vi "Wiimote Parse Extension Controller.vi"(8 "error in":errorcluster, 11 "pReportBuffer in":u8[](array[numeric]) format="%02x") -> (0 "error out":errorcluster, 1 "Nunchuk Buttons out":T1, 2 "Nunchuk Acceleration Raw out":T2, 3 "Nunchuk Analog Stick out":T3)   [LabVIEW 2011, in "Wiimote.lvlib"]
uses:
  Wiimote.lvlib
  Wiimote Point.ctl
  Wiimote Acceleration.ctl
  Nunchuk Buttons.ctl
panel:
  in  "Buttons In":T1
  in  "Acceleration In":T2
  in  "Analog Stick In":T3
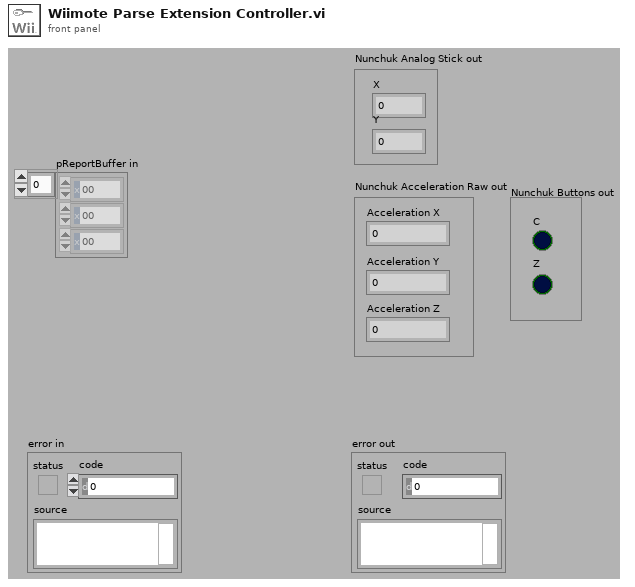
[diagram p1: front panel]
types:
  T1 = typedef "Wiimote.lvlib/Nunchuk Buttons.ctl" = cluster{"C":bool, "Z":bool}
  T2 = typedef "Wiimote.lvlib/Wiimote Acceleration.ctl" = cluster{"Acceleration X":dbl, "Acceleration Y":dbl, "Acceleration Z":dbl}
  T3 = typedef "Wiimote.lvlib/Wiimote Point.ctl" = cluster{"X":u16, "Y":u16}
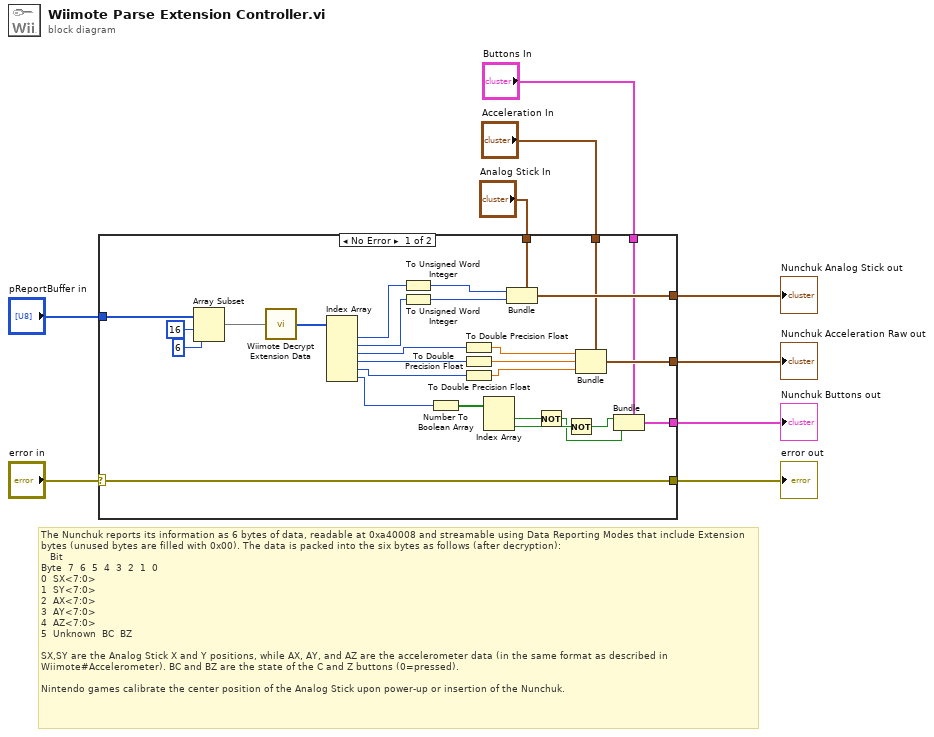
[diagram p0: block diagram]
diagram:
  # "The Nunchuk reports its information as 6 bytes of data, readable at 0xa40008 and streamable using Data Reporting Modes that include Extension bytes (unused bytes are filled with 0x00). The data is packed into the six bytes as follows (after decryption):\n  \tBit\nByte \t7 \t6 \t5 \t4 \t3 \t2 \t1 \t0\n0 \tSX<7:0>\n1 \tSY<7:0>\n2 \tAX<7:0>\n3 \tAY<7:0>\n4 \tAZ<7:0>\n5 \tUnknown \tBC \tBZ\n\nSX,SY are the Analog Stick X and Y positions, while AX, AY, and AZ are the accelerometer data (in the same format as described in Wiimote#Accelerometer). BC and BZ are the state of the C and Z buttons (0=pressed).\n\nNintendo games calibrate the center position of the Analog Stick upon power-up or insertion of the Nunchuk."
  n1 = case shown="No Error" "error in" {
    selector: "error in" -> [w37 w38]
    tunnel: [w37 w38] -> w8
    tunnel: "pReportBuffer in" -> [w34 _]
    tunnel: "Analog Stick In" -> [w31 _]
    tunnel: [w26 _] -> w5
    tunnel: "Acceleration In" -> [w22 _]
    tunnel: [w18 _] -> w3
    tunnel: "Buttons In" -> [w15 _]
    tunnel: [w12 _] -> w1
    frame No Error {
      n2 = Array Subset(array=w34, index=16, length=6) -> (w33:u8[])
      n3 = call "Wiimote Decrypt Extension Data.vi"("Encrypted Data in"=w33) -> ("Decrypted Data out"=w32:u8[])
      n4 = Index Array(array=w32) -> (element #1=w30:u8, element #2=w28:u8, element #3=w25:u8, element #4=w24:u8, element #5=w23:u8, element #6=w16:u8)  [unwired: 6 in]
      n5 = To Unsigned Word Integer(number=w30) -> (unsigned 16bit integer=w29:u16)
      n6 = To Unsigned Word Integer(number=w28) -> (unsigned 16bit integer=w27:u16)
      n7 = Number To Boolean Array(number=w16) -> (Boolean array=w17:bool[])
      n8 = To Double Precision Float(number=w25) -> (double precision float=w21:dbl)
      n9 = To Double Precision Float(number=w24) -> (double precision float=w20:dbl)
      n10 = To Double Precision Float(number=w23) -> (double precision float=w19:dbl)
      n11 = Index Array(array=w17) -> (element #1=w14:bool, element #2=w13:bool)  [unwired: 2 in]
      n12 = Bundle(cluster=w31, "X"=w29, "Y"=w27) -> (w26:T3)
      n13 = Not(x=w14) -> (.not. x?=w10:bool)
      n14 = Not(x=w13) -> (.not. x?=w11:bool)
      n15 = Bundle(cluster=w22, "Acceleration X"=w21, "Acceleration Y"=w20, "Acceleration Z"=w19) -> (w18:T2)
      n16 = Bundle(cluster=w15, "C"=w11, "Z"=w10) -> (w12:T1)
    }
    frame Error {
    }
  }
  "error out" <- w8
  "Nunchuk Analog Stick out" <- w5
  "Nunchuk Acceleration Raw out" <- w3
  "Nunchuk Buttons out" <- w1
